vi "Transmitter.vi"() -> ()   [LabVIEW 2015]
doc: "This example <B>requires the Modulation Toolkit</B>.\n\nApplies PSK (Phase Shift Keyed Modulation) to a PN sequence for USRP-based transmission. Continuously transmits a repeating message with a length determined by the PN Sequence Order parameter. \n\nThis example is paired with the example \"niUSRP Ex PSK Rx.vi\", which allows you to establish a Tx / Rx link between two separate USRPs. \n\nTo establish a Tx / Rx link between two USRPs:\n1) Ensure that the Tx and Rx example VIs have matching parameters for Modulation Scheme (M-Ary), Carrier Frequency, and Symbol Rate. Specify the Symbol Rate by setting the combination of the IQ Sampling Rate and the Number of Samples per Symbol parameters.\n2) Choose an IQ Sample Rate that enables sufficient Rx bandwidth.\n3) Set the Tx and / or Rx gain to ensure a sufficient signal to noise ratio on the Receive side. Note: applying too much gain can result in clipping.\n4) Choose a sufficient acquisition frame length to enable the demodulator to lock to the transmitted signal. National Instruments recommends that the acquired frame contain a number of symbols that is at least 20 * M-Ary of the modulation scheme. \n5) Ensure that the Reset Demodulator control is set to True until a solid lock is established. \n6) Install antennas and attenuators that efficiently operate at the carrier frequency you choose."
uses:
  <vilib>/addons/Modulation/Digital/General/MT Generate PSK System Parameters(M).vi
  <instrlib>/niUSRP/niUSRP Write Tx Data (CDB Cluster).vi
  <vilib>/addons/Modulation/niDMT.lvlib
panel:
  out "Complex Waveform":dbl[](graph)
  out "No. of bits/symbol":dbl
  in  "Enabled Channel":string(combo)="0"
  in  "Antenna":string(combo)="TX1"
  in  "Gain [dB]":dbl=12.0 format="%#.6p"
  in  "Carrier\nFrequency [Hz]":dbl=915000000.0 format="%#.6p"
  in  "IQ Sampling\nRate [S/sec]":dbl=500000.0 format="%#.6p"
  in  "device name":refnum<k15>="192.168.10.5"
  in  "Choose a PSK Format":enum32{"BPSK", "QPSK"}(tab)=enum."QPSK" caption="PSK"
  in  "BPSK System Parameters":T1={"Samples per Symbol"=8, "symbol map"=[]} {"symbol map" format="%.3f"}
  in  "QPSK System Parameters":T1={"Samples per Symbol"=8, "symbol map"=[]} {"symbol map" format="%.3f"}
  out "Frame samples":i32=4092
  in  "PN Sequence Order":i32=10
  in  "filter parameters":T2={"Alpha"=0.5, "Filter Length"=6, "TX Filter"=enum."Root Raised Cos"} {"Alpha" format="%.2f"}
  out "Symbol Rate\n[symbols/sec]":dbl=500000.0 format="%#.6p"
  in  "stop":bool
  out "Constellation Graph":T3(graph) caption="Tx Signal Constellation"
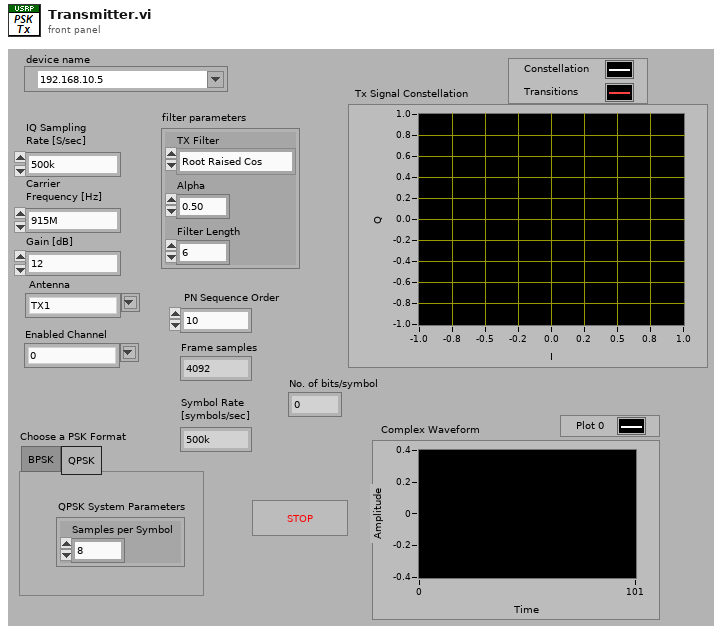
[diagram p1: front panel]
types:
  T1 = cluster{"Samples per Symbol":i32, "symbol map":cdb[]}
  T2 = cluster{"Alpha":dbl, "Filter Length":i32, "TX Filter":enum16{"none", "Raised Cosine", "Root Raised Cos", "Gaussian"}}
  T3 = cluster{"constellation":dbl[], "oversampled data":dbl[]}[]
  T4 = enum32{"PN sequence", "user-defined pattern", "Read from file"}
  T5 = cluster{"samples per symbol (16)":i32, "symbol map":cdb[], "differential PSK":enum16{"disable", "enable"}, "PSK type":u16}
  T6 = typedef "niAMT.lvlib/Complex Data Waveform.ctl" = cluster{"t0":dbl, "dt":dbl, "Y":cdb[]}
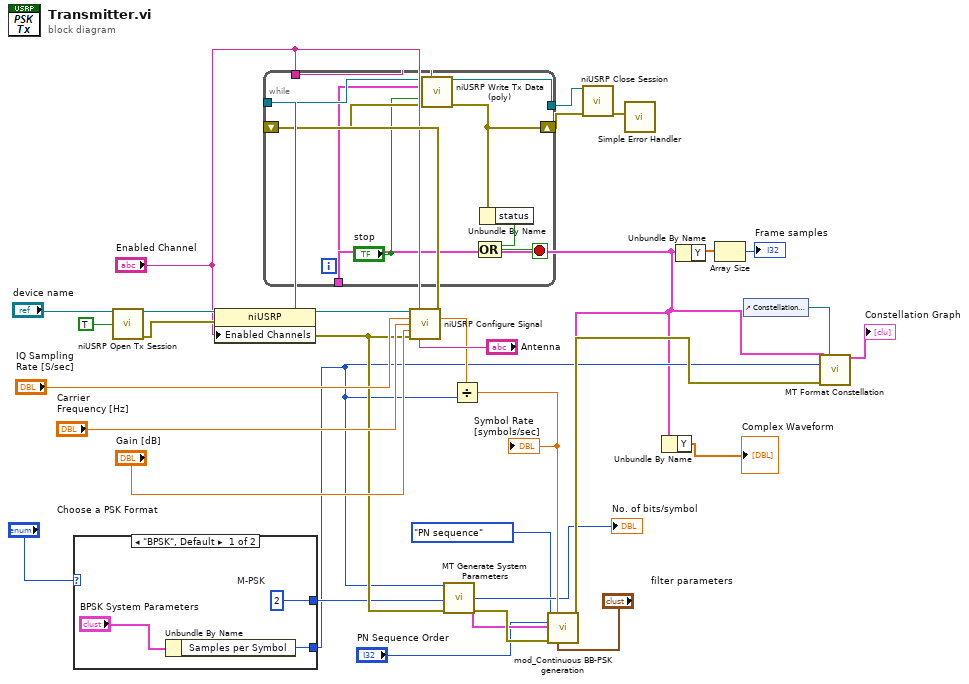
[diagram p0: block diagram]
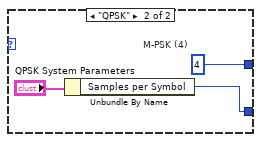
[diagram p2: hidden frame]
diagram:
  n1 = case shown="\"BPSK\", Default" "Choose a PSK Format" {
    tunnel: [w36 w38] -> w6
    tunnel: [w37 w40] -> w7
    frame "BPSK", Default {
      w37 = 2  # M-PSK
      n2 = Unbundle By Name("BPSK System Parameters") -> ("Samples per Symbol"=w36:i32)
    }
    frame "QPSK" {
      w40 = 4  # M-PSK (4)
      n3 = Unbundle By Name("QPSK System Parameters") -> ("Samples per Symbol"=w38:i32)
    }
  }
  n4 = call <instrlib>:"niUSRP Open Tx Session.vi"("device names"="device name", "reset"=TRUE) -> ("session handle out"=w15:refnum<k15>, "error out"=w14:errorcluster)  [unwired: 12 in]
  n5 = property class="niUSRP"(reference=w15, error in=w14, "Enabled Channels"="Enabled Channel") -> (reference out=w13:refnum<k15>, error out=w12:errorcluster)
  n6 = call <instrlib>:"niUSRP Configure Signal.vi"("session handle"=w13, "channel list"="Enabled Channel", "IQ rate"="IQ Sampling\nRate [S/sec]", "carrier frequency"="Carrier\nFrequency [Hz]", "gain"="Gain [dB]", "error in (no error)"=w12, "active antenna"="Antenna") -> ("session handle out"=w18:refnum<k15>, "coerced IQ rate"=w16:dbl, "error out"=w17:errorcluster)  [unwired: 4 in, 2 out]
  n7 = call-poly <vilib>:"MT Generate System Parameters.vi"("samples per symbol (16)"=w6, "M-PSK (4)"=w7, "error in (no error)"=w12) -> ("PSK system parameters"=w29:T5, "bits per symbol"=→"No. of bits/symbol":i32, "error out"=w30:errorcluster)  [unwired: 10 in]
  n8 = Divide(x=w16, y=w6) -> (x/y=w28:dbl)
  "Symbol Rate\n[symbols/sec]" <- w28
  n9 = call <vilib>:"mod_Continuous BB-PSK generation.vi"("bit stream type"=T4."PN sequence", "Symbol Rate, Hz"=w28, "Custom-PSK Parameters"=w29, "PN Sequence Order"="PN Sequence Order", "error in (no error)"=w30, "filter parameters"="filter parameters") -> ("output complex waveform"=w4:T6, "error out"=w9:errorcluster)  [unwired: 7 in, 1 out]
  n10 = while {
    tunnel: [w46] -> w26
    tunnel: w18 -> [w49]
    shift-right: [w41] -> w27
    shift-left: w17 -> [w47]
    tunnel: w4 -> [w48]
    tunnel: "Enabled Channel" -> [w42]
    stop <- w45 stop-if-true
    n11 = call-poly <instrlib>:"niUSRP Write Tx Data (poly).vi"("session handle"=w49, "channel list"=w42, "data"=w48, "end of data?"="stop", "error in (no error)"=w47) -> ("session handle out"=w46:refnum<k15>, "error out"=w41:errorcluster)  [unwired: 9 in]
    n12 = Unbundle By Name(w41) -> ("status"=w44:bool)
    n13 = Compound Arithmetic op=OR(w44, "stop") -> (w45:bool)
  }
  n14 = call <instrlib>:"niUSRP Close Session.vi"("session handle"=w26, "error in (no error)"=w27) -> ("error out"=w25:errorcluster)  [unwired: 13 in]
  n15 = call <vilib>:"Simple Error Handler.vi"("error in (no error)"=w25) -> ()  [unwired: 4 in, 5 out]
  n16 = Unbundle By Name(w4) -> ("Y"=→"Complex Waveform":cdb[])
  n17 = Unbundle By Name(w4) -> ("Y"=w32:cdb[])
  n18 = Array Size(array=w32) -> (size(s)=→"Frame samples":i32)
  n19 = control-ref of="Constellation Graph"() -> (w34:refnum<vi>)
  n20 = call <vilib>:"MT Format Constellation.vi"("waveform"=w4, "constellation reference"=w34, "samples per symbol"=w6, "error in (no error)"=w9) -> ("constellation graph"=→"Constellation Graph":T3)  [unwired: 10 in, 1 out]
